vi "Main Tree _ Click Event Pharse(position).vi"(8 "error in":errorcluster caption="错误输入", 10 "坐标":T1, 11 "Ref.Tree Ref":refnum<vi>) -> (0 "error out":errorcluster caption="错误输出", 1 "cmd?":bool, 2 "LocalData":variant, 3 "LocalEvent":string)   [LabVIEW 2016]
uses:
  <vilib>/Utility/miscctls.llb/LVPoint32TypeDef.ctl
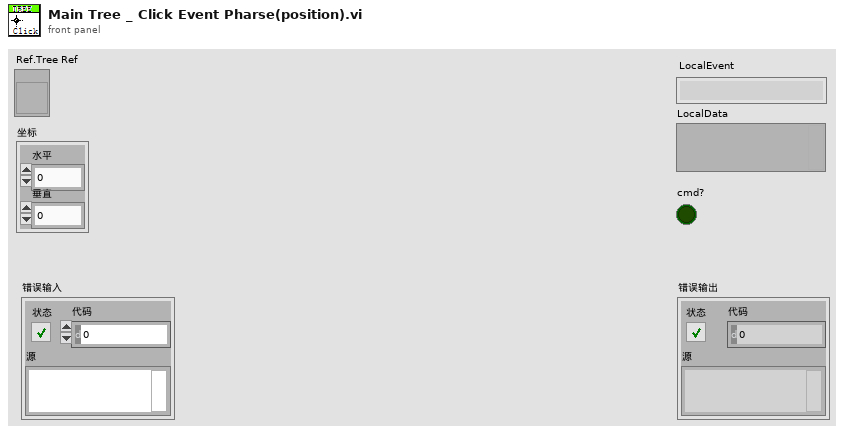
[diagram p1: front panel]
types:
  T1 = typedef "LVPoint32TypeDef.ctl" = cluster{"Horizontal":i32, "Vertical":i32}
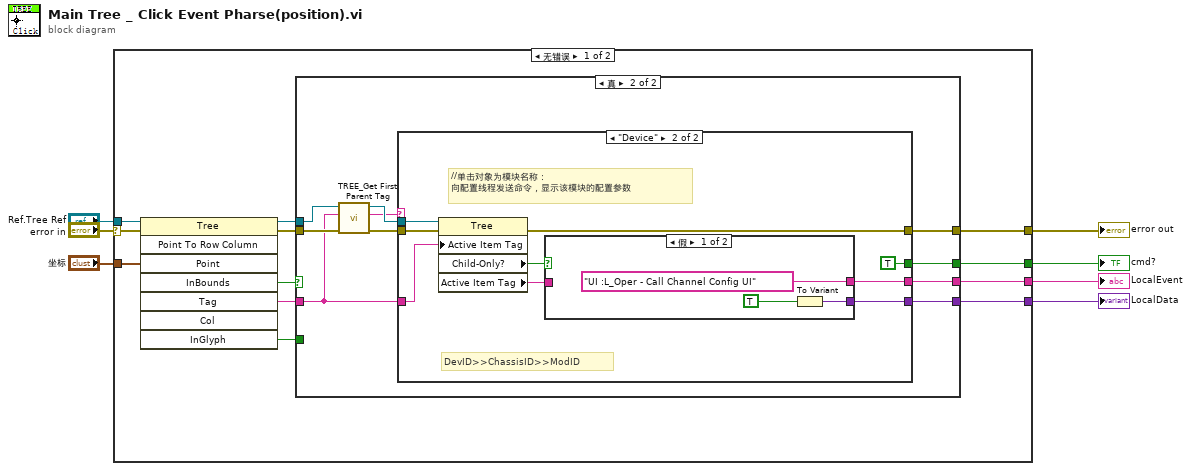
[diagram p0: block diagram]
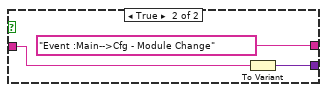
[diagram p4: hidden frame]
diagram:
  n1 = case shown="无错误" "error in" {
    selector: "error in" -> [w16 w47]
    tunnel: [w13 w47] -> w6
    tunnel: "Ref.Tree Ref" -> [w19 _]
    tunnel: "坐标" -> [w18 _]
    tunnel: [w17 _] -> w3
    tunnel: [w14 _] -> w2
    tunnel: [w12 _] -> w1
    frame No Error {
      n2 = invoke class="Tree" method="Point To Row Column"(reference=w19, error in=w16, "Point"=w18) -> (reference out=w11:refnum<vi>, error out=w15:errorcluster, "InBounds"=w9:bool, "Tag"=w10:string, "InGlyph"=w8:bool)  [unwired: 5 in, 3 out]
      n3 = case shown="真" w9 {
        tunnel: w10 -> [_ w23]
        tunnel: [_ w29] -> w17
        tunnel: w15 -> [w20 w27]
        tunnel: [_ w21] -> w14
        tunnel: [w20 w28] -> w13
        tunnel: [_ w30] -> w12
        tunnel: w11 -> [_ w25]
        tunnel: w8 -> [_ _]
        frame False {
        }
        frame True {
          n4 = call "TREE_Get First Parent Tag.vi"("error in"=w27, "tag in"=w23, "Tree Ref"=w25) -> ("error out"=w26:errorcluster, "tag out"=w22:string, "Tree Ref"=w24:refnum<vi>)  [unwired: 6 in]
          n5 = case shown="\"Device\"" w22 {
            tunnel: [_ w36] -> w30
            tunnel: w26 -> [w31 w40]
            tunnel: w24 -> [_ w39]
            tunnel: [_ TRUE ("Child-Only?")] -> w29
            tunnel: w23 -> [_ w38]
            tunnel: [w31 w37] -> w28
            tunnel: [_ w33] -> w21
            frame "假", Default {
            }
            frame "Device" {
              # "DevID>>ChassisID>>ModID"
              # "//单击对象为模块名称：\n向配置线程发送命令，显示该模块的配置参数"
              n6 = property class="Tree"(reference=w39, error in=w40, "Active Item Tag"=w38) -> (error out=w37:errorcluster, "Child-Only?"=w34:bool, "Active Item Tag"=w32:string)  [unwired: 1 out]
              n7 = case shown="假" w34 {
                tunnel: ["UI :L_Oper - Call Channel Config UI" ("正则表达式") "Event :Main-->Cfg - Module Change" ("正则表达式")] -> w36
                tunnel: [w41 w44] -> w33
                tunnel: w32 -> [_ w45]
                frame False {
                  n8 = To Variant(anything=TRUE) -> (Variant=w41:variant)
                }
                frame True {
                  n9 = To Variant(anything=w45) -> (Variant=w44:variant)
                }
              }
            }
          }
        }
      }
    }
    frame Error {
    }
  }
  "error out" <- w6
  "LocalEvent" <- w1
  "LocalData" <- w2
  "cmd?" <- w3
